vi "Configure TS DAC Relays.vi"(8 "error in":errorcluster, 11 "LNG Boiling Test Stand in":refnum<class "LNG Boiling Test Stand.lvclass">) -> (0 "error out":errorcluster, 3 "LNG Boiling Test Stand out":refnum<class "LNG Boiling Test Stand.lvclass">)   [LabVIEW 2019, in "Test Stands.lvlib" / "LNG Boiling Test Stand.lvclass"]
uses:
  LNG Boiling Test Stand.lvclass
  LNG Boiling Test Stand.lvclass/LNG Boiling Test Stand.ctl
  <vilib>/DAQmx/create/channels.llb/DAQmx Create Channel (AO-Voltage-Basic).vi
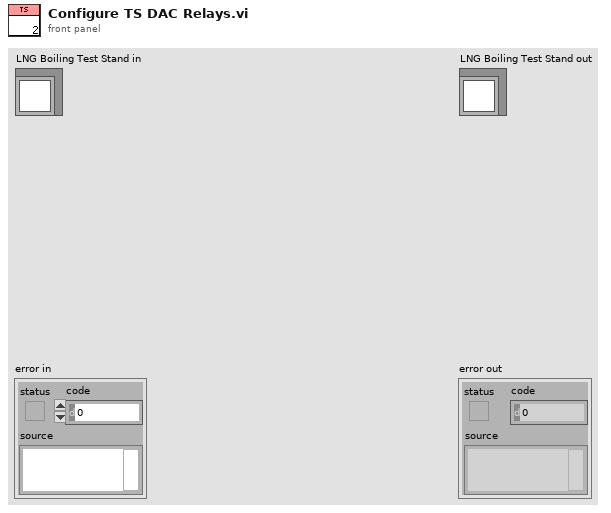
[diagram p1: front panel]
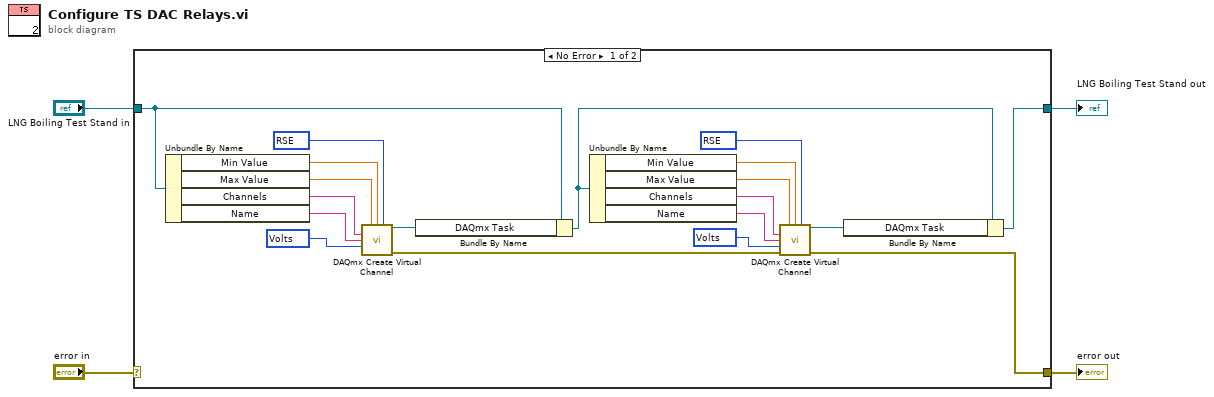
[diagram p0: block diagram]
diagram:
  n1 = case shown="No Error" "error in" {
    selector: "error in" -> [_ w25]
    tunnel: [w5 w25] -> w3
    tunnel: [w7 w24] -> w1
    tunnel: "LNG Boiling Test Stand in" -> [w17 w24]
    frame No Error {
      w9 = 10083 items=["Default"=-1, "RSE"=10083, "Differential"=10106, "Pseudodifferential"=12529] ("output terminal configuration")
      w10 = 10348 items=["Volts"=10348, "From Custom Scale"=10065] ("units")
      w18 = 10083 items=["Default"=-1, "RSE"=10083, "Differential"=10106, "Pseudodifferential"=12529] ("output terminal configuration")
      w19 = 10348 items=["Volts"=10348, "From Custom Scale"=10065] ("units")
      n2 = Unbundle By Name(w17) -> ("Min Value"=w20:dbl, "Max Value"=w21:dbl, "Channels"=w22:string, "Name"=w23:string)
      n3 = call-poly <vilib>:"DAQmx Create Virtual Channel.vi"("maximum value"=w21, "minimum value"=w20, "output terminal configuration"=w18, "physical channels"=w22, "name to assign"=w23, "units"=w19) -> ("task out"=w16:refnum<k21>, "error out"=w6:errorcluster)  [unwired: 8 in]
      n4 = Bundle By Name(cluster=w17, "DAQmx Task"=w16) -> (w15:refnum<class "LNG Boiling Test Stand.lvclass">)
      n5 = Unbundle By Name(w15) -> ("Min Value"=w11:dbl, "Max Value"=w12:dbl, "Channels"=w13:string, "Name"=w14:string)
      n6 = call-poly <vilib>:"DAQmx Create Virtual Channel.vi"("maximum value"=w12, "minimum value"=w11, "output terminal configuration"=w9, "physical channels"=w13, "name to assign"=w14, "units"=w10, "error in"=w6) -> ("task out"=w8:refnum<k21>, "error out"=w5:errorcluster)  [unwired: 7 in]
      n7 = Bundle By Name(cluster=w15, "DAQmx Task"=w8) -> (w7:refnum<class "LNG Boiling Test Stand.lvclass">)
    }
    frame Error {
    }
  }
  "error out" <- w3
  "LNG Boiling Test Stand out" <- w1
